vi "Create SSL Client Socket.vi"(8 "error in (no error)":errorcluster, 11 "SSL Client Ctx in":refnum<class "SSL Client Context.lvclass">) -> (0 "error out":errorcluster, 2 "SSL Client Socket":refnum<class "SSL Client Socket.lvclass">, 3 "SSL Client Ctx out":refnum<class "SSL Client Context.lvclass">)   [LabVIEW 2013, in "OpenSSL Socket.lvlib" / "SSL Client Context.lvclass"]
uses:
  SSL Client Context.lvclass
  SSL Client Socket/SSL Client Socket.lvclass
  SSL Context/SSL Context.lvclass/SSL Context.ctl
  Secure Socket/SSL Socket.lvclass/SSL Socket.ctl
  SSL Context/Read SSL Context.vi
  Secure Socket/Write BIO.vi
  SSL_Lib/SSL-Context/SSL-Context.lvclass
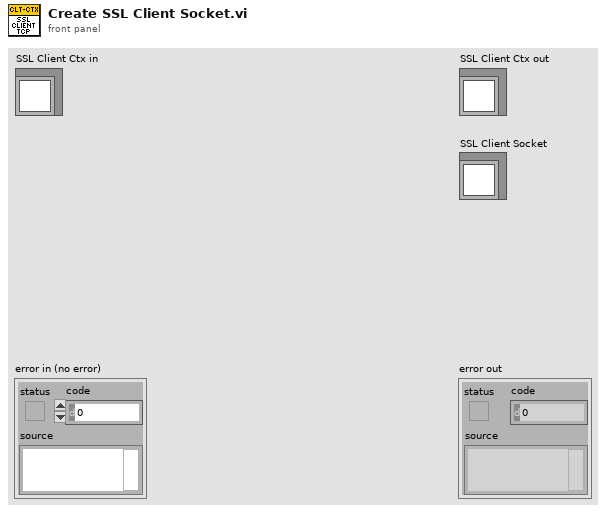
[diagram p1: front panel]
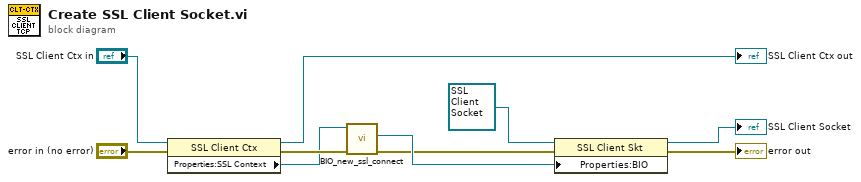
[diagram p0: block diagram]
diagram:
  n1 = property class="SSL Client Ctx"(reference="SSL Client Ctx in", error in="error in (no error)") -> (reference out=→"SSL Client Ctx out":refnum<class "SSL Client Context.lvclass">, error out=w3:errorcluster, "Properties:SSL Context"=w2:refnum<class "SSL-Context.lvclass">)
  n2 = call "BIO_new_ssl_connect.vi"("error in (no error)"=w3, "SSL-Context in"=w2) -> ("error out"=w1:errorcluster, "BIO out"=w4:refnum<class "BIO.lvclass">)  [unwired: 7 in, 1 out]
  n3 = property class="SSL Client Skt"(reference=refnum<class "SSL Client Socket.lvclass"> refnum ("SSL Client Socket"), error in=w1, "Properties:BIO"=w4) -> (reference out=→"SSL Client Socket":refnum<class "SSL Client Socket.lvclass">, error out=→"error out":errorcluster)
